vi "init data.vi"(2 "descr":string) -> (16 "nomValue":T1)   [LabVIEW 2014, in "X DIM conditions.xctl"]
uses:
  X DIM conditions.xctl
  CS_Core/CSSystem/CoreDefs/CoreDefs.rawDataType.ctl
  CS_Core/CSSystem/CoreLib/CoreLib.string 2 byte array.vi
  CS_Core/CSSystem/CoreLib/CoreLib.int 2 byte array.vi
  CS_Core/CSSystem/CoreLib/CoreLib.int array 2 byte array.vi
  CS_Core/CSSystem/CoreLib/CoreLib.short 2 byte array.vi
  CS_Core/CSSystem/CoreLib/CoreLib.short array 2 byte array.vi
  CS_Core/CSSystem/CoreLib/CoreLib.double 2 byte array.vi
  CS_Core/CSSystem/CoreLib/CoreLib.double array 2 byte array.vi
  CS_Core/CSSystem/CoreLib/CoreLib.float 2 byte array.vi
  CS_Core/CSSystem/CoreLib/CoreLib.float array 2 byte array.vi
  CS_Core/CSSystem/CoreLib/CoreLib.lvlib
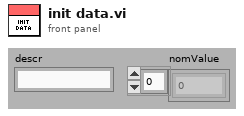
[diagram p1: front panel]
types:
  T1 = typedef "CoreDefs.rawDataType.ctl" = i8[]
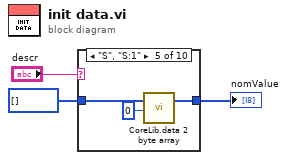
[diagram p0: block diagram]
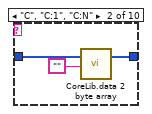
[diagram p3: hidden frame]
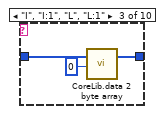
[diagram p4: hidden frame]
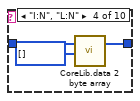
[diagram p5: hidden frame]
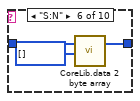
[diagram p6: hidden frame]
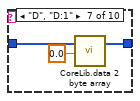
[diagram p7: hidden frame]
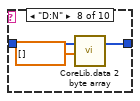
[diagram p8: hidden frame]
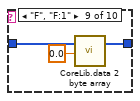
[diagram p9: hidden frame]
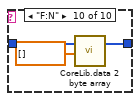
[diagram p10: hidden frame]
diagram:
  n1 = case shown="\"S\", \"S:1\"" "descr" {
    tunnel: [w4 w6 w10 w13 w16 w19 w22 w25 w28 w31] -> w2
    tunnel: T1 [] ("byteArray out") -> [w4 w5 w8 w11 w14 w17 w20 w23 w26 w29]
    frame Default {
    }
    frame "C", "C:1", "C:N" {
      n2 = call-poly "CoreLib.data 2 byte array.vi"("byteArray"=w5, "string"="") -> ("byteArray out"=w6:T1)  [unwired: 17 in]
    }
    frame "I", "I:1", "L", "L:1" {
      n3 = call-poly "CoreLib.data 2 byte array.vi"("byteArray"=w8, "i32"=0) -> ("byteArray out"=w10:T1)  [unwired: 17 in]
    }
    frame "I:N", "L:N" {
      n4 = call-poly "CoreLib.data 2 byte array.vi"("byteArray"=w11, "[i32]"=i32[] []) -> ("byteArray out"=w13:T1)  [unwired: 17 in]
    }
    frame "S", "S:1" {
      n5 = call-poly "CoreLib.data 2 byte array.vi"("byteArray"=w14, "i16"=i16 0) -> ("byteArray out"=w16:T1)  [unwired: 17 in]
    }
    frame "S:N" {
      n6 = call-poly "CoreLib.data 2 byte array.vi"("byteArray"=w17, "[i16]"=i16[] []) -> ("byteArray out"=w19:T1)  [unwired: 17 in]
    }
    frame "D", "D:1" {
      n7 = call-poly "CoreLib.data 2 byte array.vi"("byteArray"=w20, "f64"=0.0) -> ("byteArray out"=w22:T1)  [unwired: 17 in]
    }
    frame "D:N" {
      n8 = call-poly "CoreLib.data 2 byte array.vi"("byteArray"=w23, "[d64]"=dbl[] []) -> ("byteArray out"=w25:T1)  [unwired: 17 in]
    }
    frame "F", "F:1" {
      n9 = call-poly "CoreLib.data 2 byte array.vi"("byteArray"=w26, "f32"=sgl 0.0) -> ("byteArray out"=w28:T1)  [unwired: 17 in]
    }
    frame "F:N" {
      n10 = call-poly "CoreLib.data 2 byte array.vi"("byteArray"=w29, "[f32]"=sgl[] []) -> ("byteArray out"=w31:T1)  [unwired: 17 in]
    }
  }
  "nomValue" <- w2
